vi "Ouit.vi"(8 "error in (no error)":errorcluster, 9 "BL":bool, 11 "FlowCtrl in":refnum<class "Station Action.lvclass">) -> (0 "error out":errorcluster, 3 "FlowCtrl out":refnum<class "Station Action.lvclass">)   [LabVIEW 2019, in "Station Action.lvclass"]
uses:
  Station Action.lvclass
  Function/IO Folder/IO_Class/IOCard.lvclass
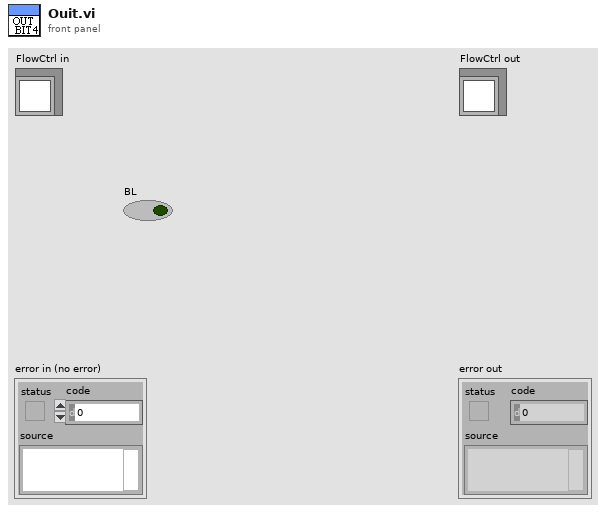
[diagram p1: front panel]
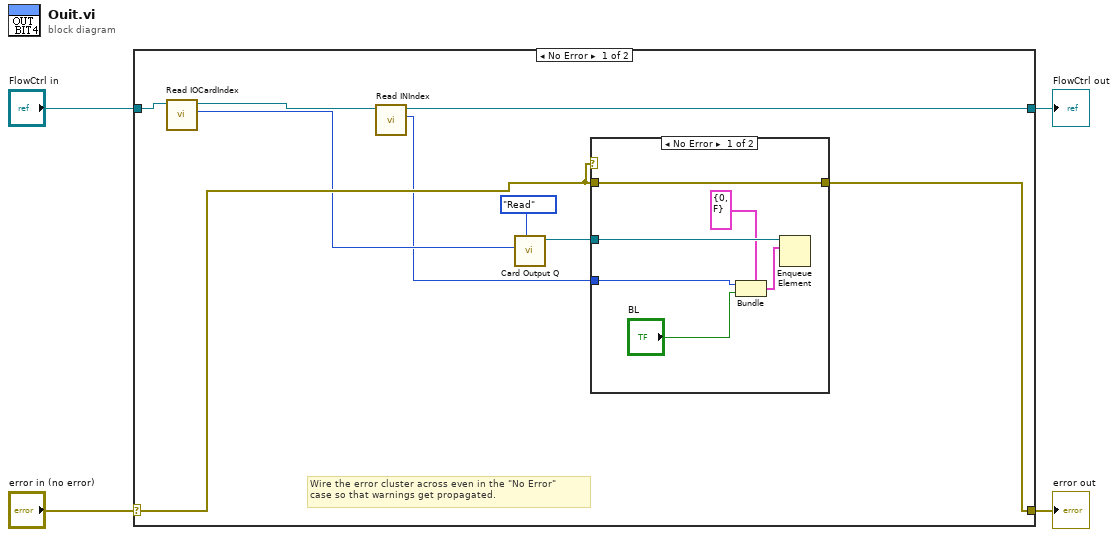
[diagram p0: block diagram]
diagram:
  n1 = case shown="No Error" "error in (no error)" {
    selector: "error in (no error)" -> [w10 w22]
    tunnel: [w9 w22] -> w3
    tunnel: [w6 w21] -> w1
    tunnel: "FlowCtrl in" -> [w13 w21]
    frame No Error {
      # "Wire the error cluster across even in the \"No Error\"\ncase so that warnings get propagated."
      n2 = call-dynamic "Read IOCardIndex.vi"("Station Action in"=w13) -> ("IOCardIndex"=w7:i32, "Station Action out"=w8:refnum<class "Station Action.lvclass">)  [unwired: 8 in, 1 out]
      n3 = call-dynamic "Read INIndex.vi"("Station Action in"=w8) -> ("INIndex"=w5:i32, "Station Action out"=w6:refnum<class "Station Action.lvclass">)  [unwired: 8 in, 1 out]
      n4 = call "Card Output Q.vi"("Action"=enum16{"Initial", "Write", "Read", "Release"}."Read", "CardIndex"=w7) -> ("Output Q Out"=w11:refnum<queue>)  [unwired: 8 in, 1 out]
      n5 = case shown="No Error" w10 {
        tunnel: w10 -> [w18 w20]
        tunnel: [w18 w20] -> w9
        tunnel: w11 -> [w19 _]
        tunnel: w5 -> [w14 _]
        frame No Error {
          n6 = Bundle(cluster=cluster{"Index":i32, "BL":bool} {"Index"=0, "BL"=FALSE} ("element"), "Index"=w14, "BL"="BL") -> (w15:cluster{"Index":i32, "BL":bool})
          n7 = Enqueue Element(queue=w19, element=w15) -> ()  [unwired: 2 in, 3 out]
        }
        frame Error {
        }
      }
    }
    frame Error {
    }
  }
  "error out" <- w3
  "FlowCtrl out" <- w1
